vi "Contents Summary Text.vi"(11 "Message":refnum<class "MSG.lvclass">) -> (2 "Contents Summary Text":string, 3 "Message":refnum<class "MSG.lvclass">)   [LabVIEW 2011, in "Messenging.lvlib" / "MSG.lvclass"]
uses:
  MSG.lvclass
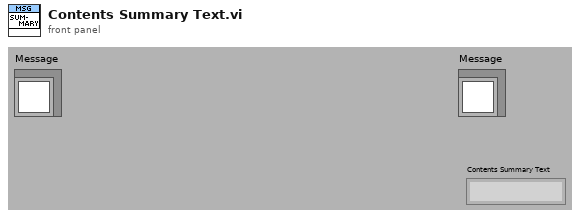
[diagram p1: front panel]
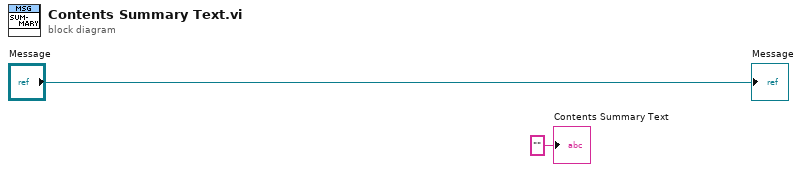
[diagram p0: block diagram]
diagram:
  "Message" <- "Message"
  "Contents Summary Text" <- "" ("Summary Text")
